vi "状态读取.vi"   [LabVIEW 2020]
uses:
  Global_Variable/Global.vi
types:
  T1 = cluster{"相机结果":dbl, "电缸位移":sgl, "工装移载位移":sgl, "1":sgl, "输入扭矩":sgl, "拉压力":sgl, "拉压力":sgl, "一点":sgl}
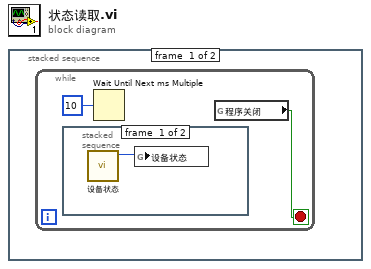
[diagram p0: block diagram]
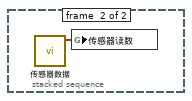
[diagram p2: hidden frame]
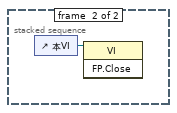
[diagram p3: hidden frame]
diagram:
  n1 = stacked-sequence {
    frame #0 {
      n2 = while {
        stop <- w1 stop-if-true
        n3 = stacked-sequence {
          frame #0 {
            n4 = call "设备状态.vi"() -> ("Status_Read"=w3:i16)  [unwired: 11 in]
            n5 = global write "Global.vi" "设备状态"(w3) -> ()
          }
          frame #1 {
            n6 = call "传感器数据.vi"() -> ("传感器读数"=w4:T1)  [unwired: 11 in]
            n7 = global write "Global.vi" "传感器读数"(w4) -> ()
          }
        }
        n8 = Wait Until Next ms Multiple(millisecond multiple=u32 10 ("毫秒倍数")) -> ()  [unwired: 1 out]
        n9 = global read "Global.vi" "程序关闭"() -> (w1:bool)
      }
    }
    frame #1 {
      n10 = control-ref of="本VI"() -> (w5:refnum<vi>)
      n11 = invoke class="VI" method="FP.Close"(reference=w5) -> ()  [unwired: 2 in, 3 out]
    }
  }
